vi "Drive_CalculateMovement.vi"(3 "error in":errorcluster, 4 "Mode":T1 items=["TurnThenStraight"], 5 "Y rel":dbl, 6 "X rel":dbl) -> (0 "error out":errorcluster, 2 "Movements":cluster{"Left":dbl, "Right":dbl}[](array[cluster]))   [LabVIEW 2009, in "Drive.lvlib"]
doc: "Calculates a sequence of movements to the specified point depending on the mode.\n\nFor TurnThenStraight mode outputs two movements - turning on spot then moving straight ahead."
uses:
  Drive.lvlib
  Drive_PositionControlMode.ctl
  Drive_Utils.lvlib
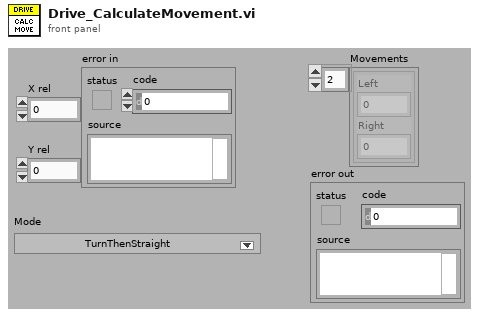
[diagram p1: front panel]
types:
  T1 = typedef "Drive.lvlib/Drive_PositionControlMode.ctl" = u16
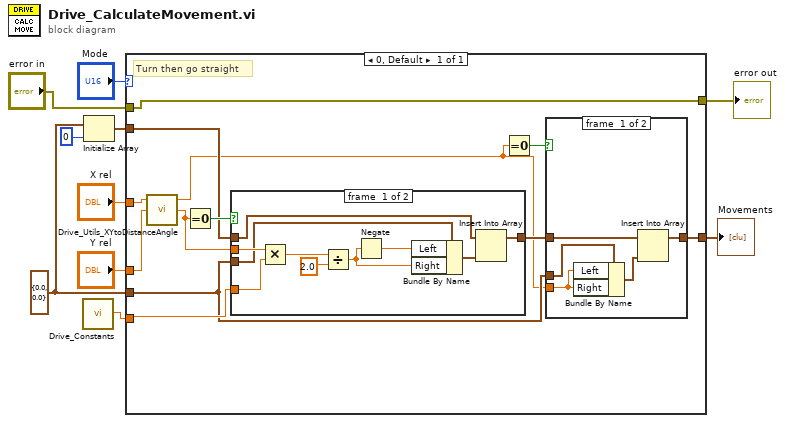
[diagram p0: block diagram]
diagram:
  w4 = cluster{"Left":dbl, "Right":dbl} {"Left"=0.0, "Right"=0.0} ("Movement")
  n1 = call "Drive_Constants.vi"() -> ("Speed convert constant"=w7:dbl)  [unwired: 23 in, 4 out]
  n2 = Initialize Array(w4, 0 ("dimension size")) -> (w3:cluster{"Left":dbl, "Right":dbl}[])
  n3 = case shown="0, Default" "Mode" {
    tunnel: "X rel" -> [w22]
    tunnel: "Y rel" -> [w21]
    tunnel: w7 -> [w20]
    tunnel: [w13] -> w6
    tunnel: w4 -> [w17]
    tunnel: w3 -> [w16]
    tunnel: "error in" -> [w11]
    tunnel: [w11] -> w1
    frame 0, Default {
      # "Turn then go straight"
      n4 = call "Drive_Utils_XYtoDistanceAngle.vi"("Y"=w21, "X"=w22) -> ("Angle (rad)"=w18:dbl, "Distance"=w12:dbl)  [unwired: 1 in, 1 out]
      n5 = Equal To 0?(x=w18) -> (x = 0?=w19:bool)
      n6 = case shown="False" w19 {
        tunnel: w18 -> [w38 _]
        tunnel: w20 -> [w37 _]
        tunnel: w17 -> [w32 _]
        tunnel: [w31 w39] -> w14
        tunnel: w16 -> [w29 w39]
        frame #0 {
          n7 = Multiply(x=w38, y=w37) -> (x*y=w36:dbl)
          n8 = Divide(x=w36, y=2.0) -> (x/y=w33:dbl)
          n9 = Negate(x=w33) -> (-x=w34:dbl)
          n10 = Bundle By Name(cluster=w32, "Left"=w34, "Right"=w33) -> (w30:cluster{"Left":dbl, "Right":dbl})
          n11 = Insert Into Array(array=w29, new element=w30) -> (w31:cluster{"Left":dbl, "Right":dbl}[])  [unwired: 1 in]
        }
        frame #1 {
        }
      }
      n12 = Equal To 0?(x=w12) -> (x = 0?=w15:bool)
      n13 = case shown="False" w15 {
        tunnel: w17 -> [w27 _]
        tunnel: w12 -> [w26 _]
        tunnel: w14 -> [w25 w28]
        tunnel: [w24 w28] -> w13
        frame #0 {
          n14 = Bundle By Name(cluster=w27, "Left"=w26, "Right"=w26) -> (w23:cluster{"Left":dbl, "Right":dbl})
          n15 = Insert Into Array(array=w25, new element=w23) -> (w24:cluster{"Left":dbl, "Right":dbl}[])  [unwired: 1 in]
        }
        frame #1 {
        }
      }
    }
  }
  "Movements" <- w6
  "error out" <- w1
